vi "Configure Trigger (Video).vi"(0 "VISA resource name":refnum<visa-resource-name>, 1 "Video Standard (0: NTSC)":u16(ring) items=["NTSC", "PAL/SECAM"], 2 "Video Polarity (0: Positive)":u16(ring) items=["Positive", "Negative"], 5 "Trigger Source (0: Channel 1)":u16(ring) items=["Channel 1", "Channel 2", "Channel 3", "Channel 4", "EXT", "EXT5"], 7 "Trigger Level (0.0 V)":dbl, 11 "error in (no error)":errorcluster, 12 "Video Sync (0: All Lines)":u16(ring) items=["All Lines", "Line", "ODD Fields", "EVEN Fields"], 13 "Video Line (1)":u32=1) -> (4 "VISA resource name out":refnum<visa-resource-name>, 15 "error out":errorcluster)   [LabVIEW 2017, in "RIGOL DS1000 Series.lvlib"]
doc: "Configures video trigger settings for an oscilloscope."
uses:
  RIGOL DS1000 Series.lvlib
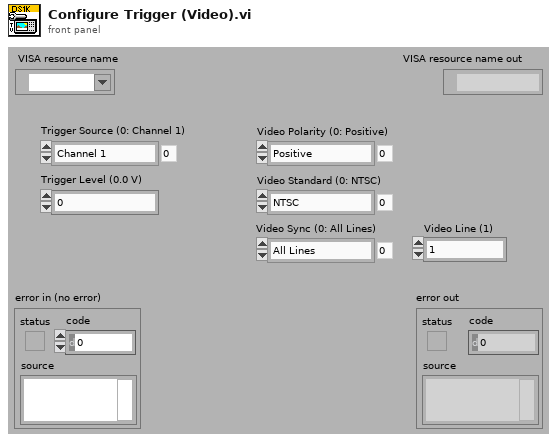
[diagram p1: front panel]
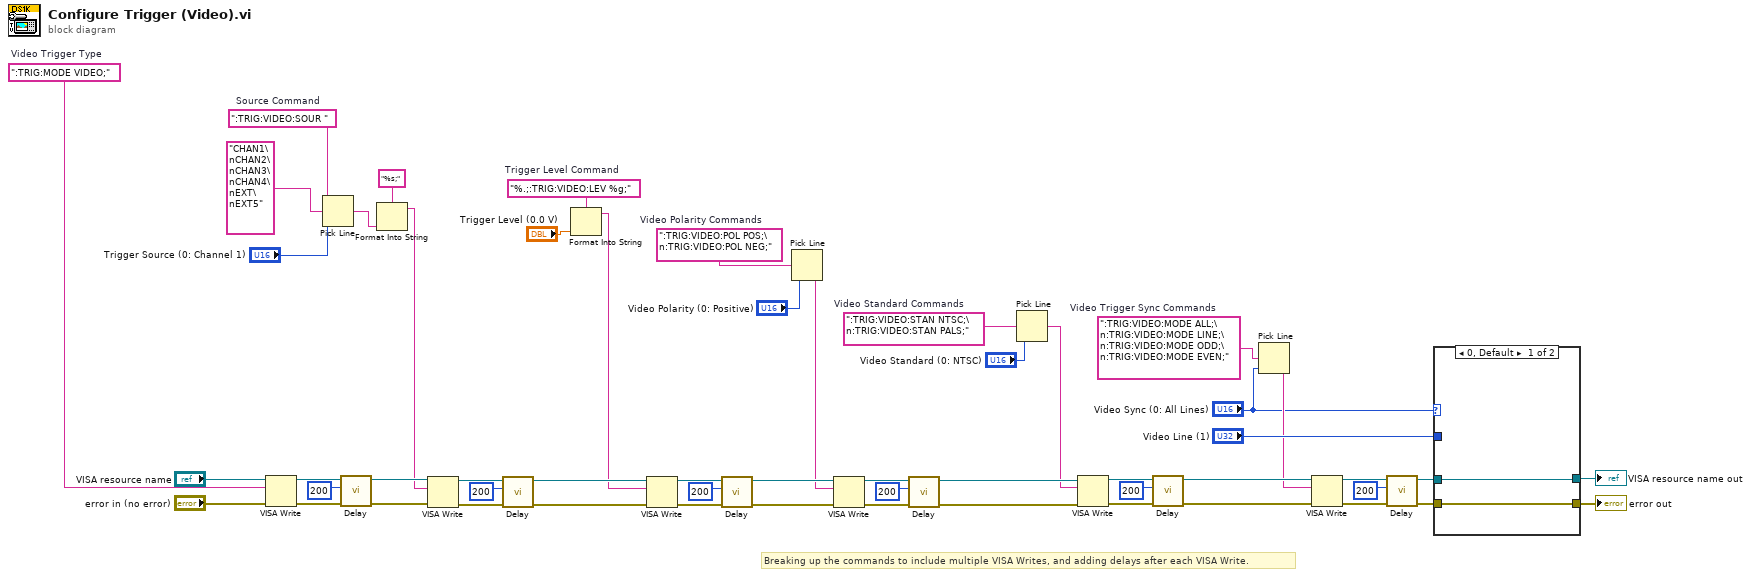
[diagram p0: block diagram]
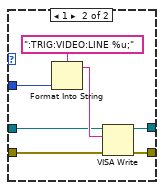
[diagram p2: hidden frame]
diagram:
  w52 = "%.;:TRIG:VIDEO:LEV %g;"  # Trigger Level Command
  w40 = ":TRIG:MODE VIDEO;"  # Video Trigger Type
  w49 = ":TRIG:VIDEO:SOUR "  # Source Command
  w53 = ":TRIG:VIDEO:POL POS;\n:TRIG:VIDEO:POL NEG;"  # Video Polarity Commands
  w5 = ":TRIG:VIDEO:MODE ALL;\n:TRIG:VIDEO:MODE LINE;\n:TRIG:VIDEO:MODE ODD;\n:TRIG:VIDEO:MODE EVEN;"  # Video Trigger Sync Commands
  w4 = ":TRIG:VIDEO:STAN NTSC;\n:TRIG:VIDEO:STAN PALS;"  # Video Standard Commands
  # "Breaking up the commands to include multiple VISA Writes, and adding delays after each VISA Write."
  n1 = VISA Write(VISA resource name="VISA resource name", write buffer=w40, error in (no error)="error in (no error)") -> (VISA resource name out=w45:refnum<visa-resource-name>, error out=w44:errorcluster)  [unwired: 1 out]
  n2 = Pick Line(string ("")=w49, multi-line string="CHAN1\nCHAN2\nCHAN3\nCHAN4\nEXT\nEXT5" ("多行字符串"), line index="Trigger Source (0: Channel 1)") -> (output string=w46:string)
  n3 = call "Delay.vi"("error in (no error)"=w44, "Delay (ms)"=u32 200, "VISA resource name"=w45) -> ("error out"=w35:errorcluster, "VISA resource name out"=w36:refnum<visa-resource-name>)  [unwired: 7 out]
  n4 = Format Into String(format string="%s;", w46) -> (resulting string=w1:string)  [unwired: 2 in, 1 out]
  n5 = VISA Write(VISA resource name=w36, write buffer=w1, error in (no error)=w35) -> (VISA resource name out=w39:refnum<visa-resource-name>, error out=w38:errorcluster)  [unwired: 1 out]
  n6 = call "Delay.vi"("error in (no error)"=w38, "Delay (ms)"=u32 200, "VISA resource name"=w39) -> ("error out"=w30:errorcluster, "VISA resource name out"=w31:refnum<visa-resource-name>)  [unwired: 7 out]
  n7 = Format Into String(format string=w52, "Trigger Level (0.0 V)") -> (resulting string=w29:string)  [unwired: 2 in, 1 out]
  n8 = VISA Write(VISA resource name=w31, write buffer=w29, error in (no error)=w30) -> (VISA resource name out=w34:refnum<visa-resource-name>, error out=w33:errorcluster)  [unwired: 1 out]
  n9 = call "Delay.vi"("error in (no error)"=w33, "Delay (ms)"=u32 200, "VISA resource name"=w34) -> ("error out"=w24:errorcluster, "VISA resource name out"=w25:refnum<visa-resource-name>)  [unwired: 7 out]
  n10 = Pick Line(multi-line string=w53, line index="Video Polarity (0: Positive)") -> (output string=w23:string)  [unwired: 1 out]
  n11 = VISA Write(VISA resource name=w25, write buffer=w23, error in (no error)=w24) -> (VISA resource name out=w28:refnum<visa-resource-name>, error out=w27:errorcluster)  [unwired: 1 out]
  n12 = call "Delay.vi"("error in (no error)"=w27, "Delay (ms)"=u32 200, "VISA resource name"=w28) -> ("error out"=w18:errorcluster, "VISA resource name out"=w19:refnum<visa-resource-name>)  [unwired: 7 out]
  n13 = Pick Line(multi-line string=w4, line index="Video Standard (0: NTSC)") -> (output string=w17:string)  [unwired: 1 out]
  n14 = VISA Write(VISA resource name=w19, write buffer=w17, error in (no error)=w18) -> (VISA resource name out=w22:refnum<visa-resource-name>, error out=w21:errorcluster)  [unwired: 1 out]
  n15 = call "Delay.vi"("error in (no error)"=w21, "Delay (ms)"=u32 200, "VISA resource name"=w22) -> ("error out"=w12:errorcluster, "VISA resource name out"=w13:refnum<visa-resource-name>)  [unwired: 7 out]
  n16 = Pick Line(multi-line string=w5, line index="Video Sync (0: All Lines)") -> (output string=w11:string)  [unwired: 1 out]
  n17 = VISA Write(VISA resource name=w13, write buffer=w11, error in (no error)=w12) -> (VISA resource name out=w16:refnum<visa-resource-name>, error out=w15:errorcluster)  [unwired: 1 out]
  n18 = call "Delay.vi"("error in (no error)"=w15, "Delay (ms)"=u32 200, "VISA resource name"=w16) -> ("error out"=w8:errorcluster, "VISA resource name out"=w10:refnum<visa-resource-name>)  [unwired: 7 out]
  n19 = case shown="0, Default" "Video Sync (0: All Lines)" {
    tunnel: "Video Line (1)" -> [_ w63]
    tunnel: w10 -> [w56 w60]
    tunnel: [w56 w58] -> w9
    tunnel: w8 -> [w55 w59]
    tunnel: [w55 w57] -> w7
    frame 0, Default {
    }
    frame 1 {
      n20 = Format Into String(format string=":TRIG:VIDEO:LINE %u;", w63) -> (resulting string=w61:string)  [unwired: 2 in, 1 out]
      n21 = VISA Write(VISA resource name=w60, write buffer=w61, error in (no error)=w59) -> (VISA resource name out=w58:refnum<visa-resource-name>, error out=w57:errorcluster)  [unwired: 1 out]
    }
  }
  "error out" <- w7
  "VISA resource name out" <- w9
